vi "Reactor.vi"() -> ()   [LabVIEW 2017]
uses:
  <vilib>/Analysis/baseanly.llb/Mean (DBL).vi
  <vilib>/Utility/file.llb/Read Delimited Spreadsheet (DBL).vi
  <vilib>/Analysis/NI_AALBase.lvlib
panel:
  in  "CTAH Set Point":sgl format="%.1f"
  in  "Mode":string(combo)
  in  "Reset IHX Controller Mode":bool
  out "Server OK":bool
  out "System Time [s]":sgl
  out "Power Output":sgl(graph)
  out "Frequency [Hz]":sgl(slide) scale=0.0..60.0
  out "Frequency [Hz]":sgl(slide) scale=0.0..60.0
  out "Frequency [Hz]":sgl(knob) scale=0.0..45.0
  out "Power [W]":sgl(slide) caption="Power Output [W]" scale=0.0..10000.0
  in  "Desired Power [W]":dbl min=0.0 max=1000.0 step=1.0 format="%.1f"
  out "WT-10":sgl format="%.1f"
  out "BT-11":sgl format="%.1f"
  out "BT-12":sgl format="%.1f"
  out "WT-13":sgl format="%.1f"
  out "CX-10":dbl format="%.1f"
  out "CX-11":dbl format="%.1f"
  out "WT-20":sgl format="%.1f"
  out "BT-21":sgl format="%.1f"
  out "WT-22":sgl format="%.1f"
  out "BT-23":sgl format="%.1f"
  out "WT-24":sgl format="%.1f"
  out "BT-25":sgl format="%.1f"
  out "WT-26":sgl format="%.1f"
  out "BT-27":sgl format="%.1f"
  out "WT-28":sgl format="%.1f"
  out "BT-29":sgl format="%.1f"
  out "BT-30":sgl format="%.1f"
  out "WT-31":sgl format="%.1f"
  out "BT-32":sgl format="%.1f"
  out "WT-33":sgl format="%.1f"
  out "BT-34":sgl format="%.1f"
  out "WT-35":sgl format="%.1f"
  out "WT-40":sgl format="%.1f"
  out "BT-41":sgl format="%.1f"
  out "WT-42":sgl format="%.1f"
  out "BT-43":sgl format="%.1f"
  out "BT-60":sgl format="%.1f"
  out "WT-61":sgl format="%.1f"
  out "WT-62":sgl format="%.1f"
  out "BT-63":sgl format="%.1f"
  out "WT-64":sgl format="%.1f"
  out "BT-65":sgl format="%.1f"
  out "BT-66":sgl format="%.1f"
  out "WT-67":sgl format="%.1f"
  out "ST-10":sgl format="%.1f"
  out "ST-11":sgl format="%.1f"
  out "ST-12":sgl[](array[numeric]) format="%.1f"
  out "ST-13":sgl format="%.1f"
  out "ST-14":sgl[](array[numeric]) format="%.1f"
  out "AT-01":sgl format="%.1f"
  out "AT-02":sgl format="%.1f"
  in  "Power Output On":bool
  in  "ACTIVATE - CTAH":bool
  in  "ACTIVATE - TCHX":bool
  in  "TCHX Frequency [Hz]":sgl min=0 max=60 step=0.1 format="%.1f"
  in  "ACTIVATE - PUMP":bool
  in  "Pump Frequency [Hz]":sgl min=0 max=45 step=0.1 format="%.1f"
  out "DHX Primary Flow\n\n\nFM-20 [kg/s]":sgl format="%.3f"
  out "Bypass Flow\n\n\nFM-30 [kg/s]":sgl format="%.3f"
  out "Primary Flow\n\n\nFM-40 [kg/s]":sgl format="%.3f"
  out "DRACS Flow\n\n\nFM-60 [kg/s]":sgl format="%.3f"
  out "System Safe":bool
  in  "Exit Profile":bool
  in  "Select Operation Mode":T1(ring) caption="Select Operation Mode2"
  out "System Loop Time (ms)":u32
  in  "Load Power Profile":bool
  in  "Dyn. Power Profile File":path
  out "CTAH Temperatures":cluster{"CTAH Outlet":dbl, "CTAH Inlet":dbl}(graph)
  out "CTAH Outlet":dbl format="%0.2f"
  out "CTAH Inlet":dbl format="%0.2f"
  out "Core Temperatures":cluster{"Heater Inlet":dbl, "Heater Outlet":dbl}(graph)
  out "Heater Outlet":dbl format="%0.2f"
  out "Heater Inlet":dbl format="%0.2f"
  out "Profile Step":i32
  out "Power Input Signal [W]":dbl
  out "Output Current 2 [A]":dbl
  out "Output Voltage 2 [V]":dbl
  out "Output Current 1 [A]":dbl
  out "Output Voltage 1 [V]":dbl
  out "Loop Period [ms]":i64
  in  "Pump Operation Mode":i32(listbox)
  in  "TCHX Operation Mode":i32(listbox)
  in  "CTAH Operation Mode":i32(listbox)
  in  "Stop Reactor Interface":bool
  # "DRACS"
  # "PRIMARY"
  # "HOT DRACS"
  # "TCHX"
  # "HOT LEG"
  # "DHX TOP"
  # "N"
  # "COLD DRACS"
  # "DHX"
  # "E"
  # "S"
  # "W"
  # "BYPASS"
  # "N"
  # "CTAH"
  # "SE"
  # "SW"
  # "HEATER"
  # "DHX BOTTOM"
  # "COLD LEG"
  # "PUMP"
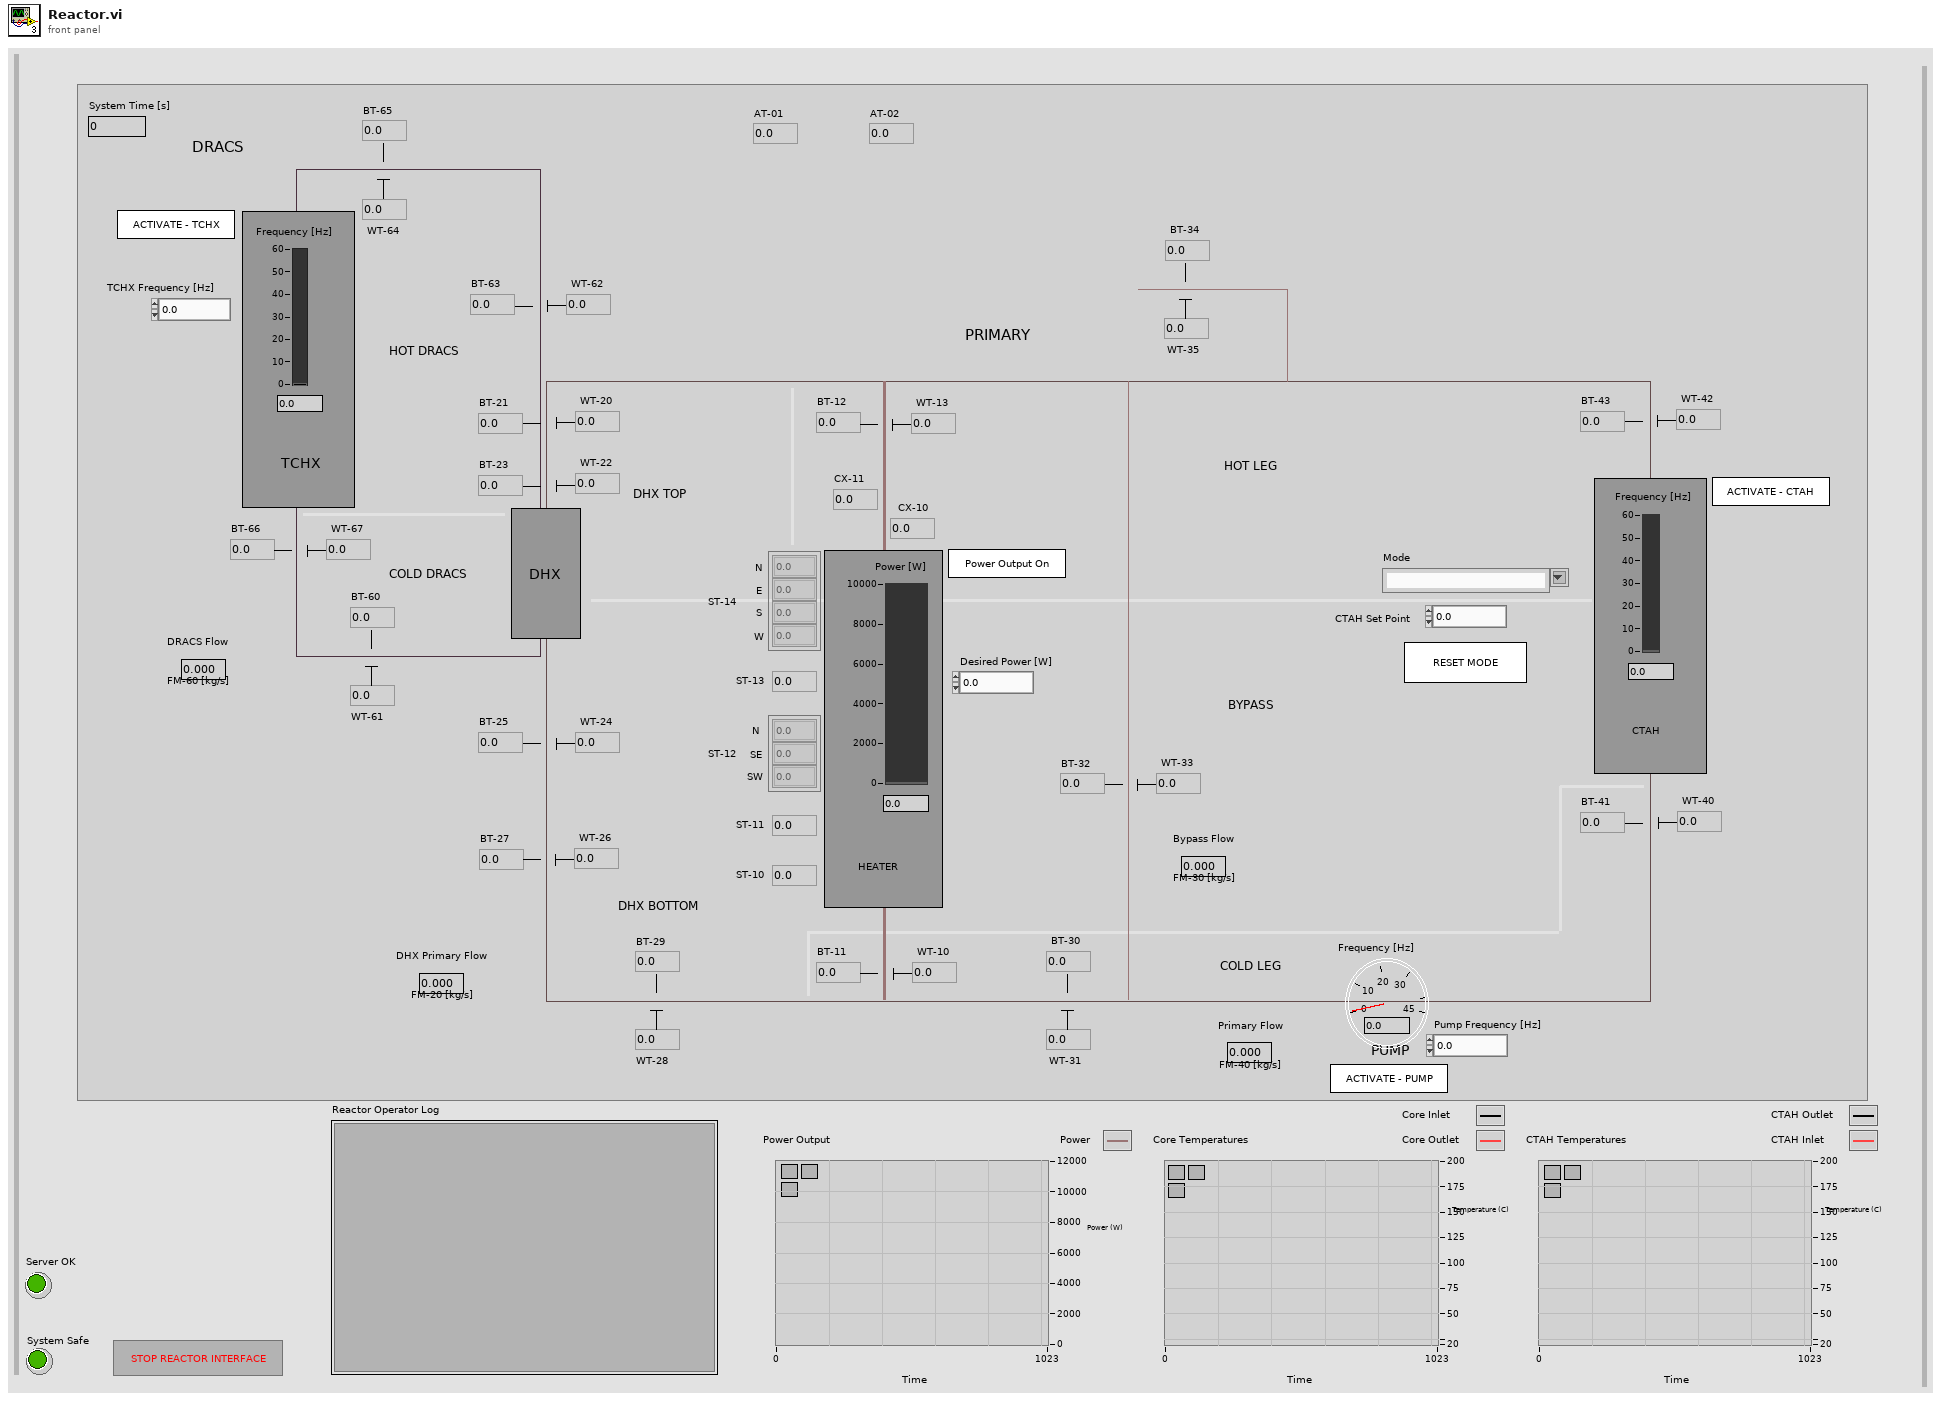
[diagram p1: front panel]
types:
  T1 = enum16{"Resistance Feedback", "Power Profile Input", "Resistance Feedback_Analog", "Power Profile Input_Analog", "Shutdown"}
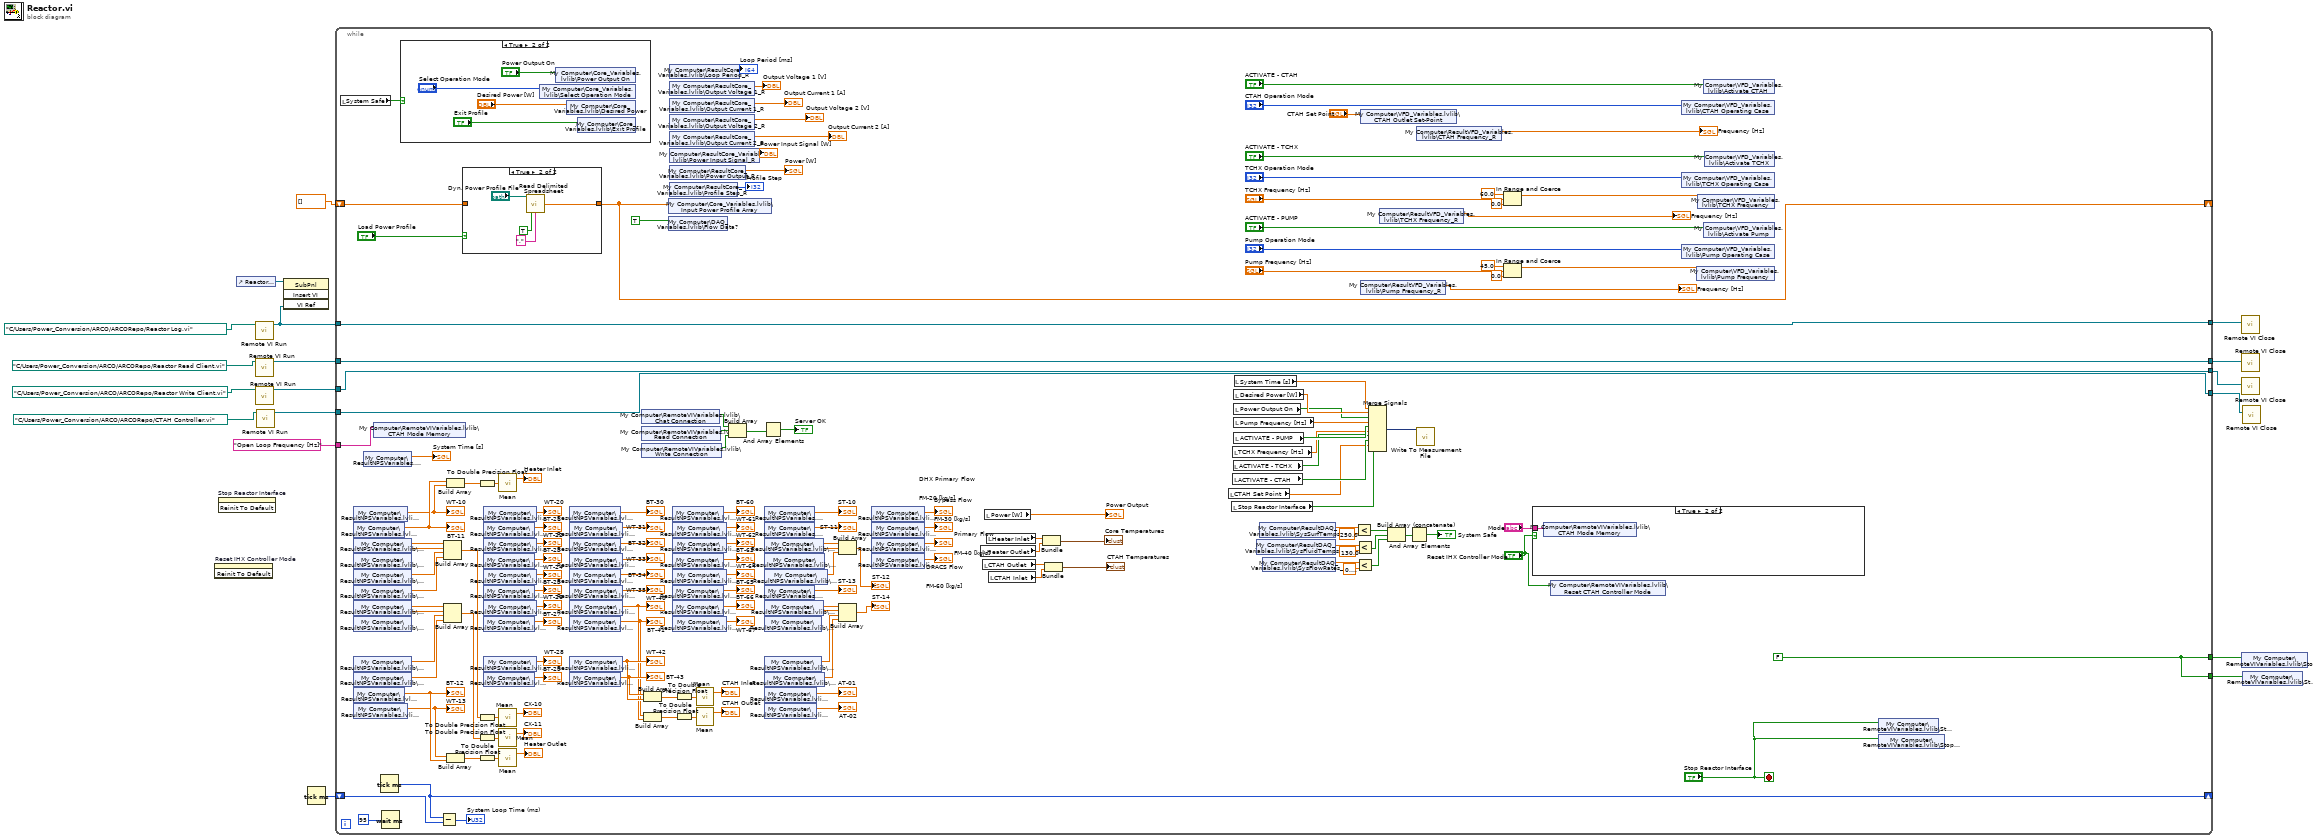
[diagram p0: block diagram]
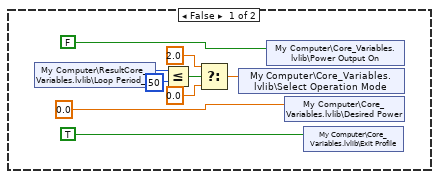
[diagram p3: hidden frame]
diagram:
  n1 = invoke on="Reset IHX Controller Mode" class="Bool" method="Reinit To Default"() -> ()  [unwired: 3 in, 3 out]
  n2 = invoke on="Stop Reactor Interface" class="Bool (strict)" method="Reinit To Default"() -> ()  [unwired: 3 in, 3 out]
  n3 = control-ref of="Reactor Operator Log"() -> (w12:refnum<vi>)
  n4 = call "Remote VI Run.vi"("VI Path"=path "C:/Users/Power_Conversion/ARCO/ARCORepo/Reactor Log.vi" ("vi path")) -> ("VI Reference"=w16:refnum<vi>)  [unwired: 10 in]
  n5 = call "Remote VI Run.vi"("VI Path"=path "C:/Users/Power_Conversion/ARCO/ARCORepo/Reactor Read Client.vi" ("vi path")) -> ("VI Reference"=w14:refnum<vi>)  [unwired: 10 in]
  n6 = call "Remote VI Run.vi"("VI Path"=path "C:/Users/Power_Conversion/ARCO/ARCORepo/Reactor Write Client.vi" ("vi path")) -> ("VI Reference"=w6:refnum<vi>)  [unwired: 10 in]
  n7 = call "Remote VI Run.vi"("VI Path"=path "C:/Users/Power_Conversion/ARCO/ARCORepo/CTAH Controller.vi" ("vi path")) -> ("VI Reference"=w3:refnum<vi>)  [unwired: 10 in]
  n8 = invoke on="Invoke Node" class="SubPnl" method="Insert VI"(reference=w12, "VI Ref"=w16) -> ()  [unwired: 2 in, 4 out]
  n9 = Tick Count (ms)() -> (millisecond timer value=w17:u32)
  n10 = while {
    shift-right: [w73] -> _
    shift-left: dbl[] [] ("Input Power Profile Array") -> [w74]
    shift-right: [w71] -> _
    shift-left: w17 -> [w72]
    tunnel: w16 -> [w53]
    tunnel: [w53] -> w15
    tunnel: w14 -> [w52]
    tunnel: [w52] -> w13
    tunnel: [w21] -> w11
    tunnel: "Open Loop Frequency [Hz]" -> [w20]
    tunnel: w6 -> [w26]
    tunnel: [w26] -> w5
    tunnel: w3 -> [w22]
    tunnel: [w22] -> w2
    tunnel: [w21] -> w1
    stop <- "Stop Reactor Interface" stop-if-true
    w21 = FALSE
    n11 = local read "System Safe"() -> (w57:bool)
    n12 = shared-variable "My Computer\\ResultNPSVariables.lvlib\\WT-10_R"() -> (w94:sgl)  [unwired: 1 in, 1 out]
    "WT-10" <- w94
    n13 = shared-variable "My Computer\\ResultNPSVariables.lvlib\\BT-11_R"() -> (w95:sgl)  [unwired: 1 in, 1 out]
    "BT-11" <- w95
    n14 = shared-variable "My Computer\\ResultNPSVariables.lvlib\\CX-10-1_R"() -> (w157:sgl)  [unwired: 1 in, 1 out]
    n15 = shared-variable "My Computer\\ResultNPSVariables.lvlib\\CX-10-2_R"() -> (w156:sgl)  [unwired: 1 in, 1 out]
    n16 = shared-variable "My Computer\\ResultNPSVariables.lvlib\\CX-10-3_R"() -> (w155:sgl)  [unwired: 1 in, 1 out]
    n17 = shared-variable "My Computer\\ResultNPSVariables.lvlib\\CX-10-4_R"() -> (w154:sgl)  [unwired: 1 in, 1 out]
    n18 = shared-variable "My Computer\\ResultNPSVariables.lvlib\\CX-11-1_R"() -> (w150:sgl)  [unwired: 1 in, 1 out]
    n19 = shared-variable "My Computer\\ResultNPSVariables.lvlib\\CX-11-2_R"() -> (w149:sgl)  [unwired: 1 in, 1 out]
    n20 = shared-variable "My Computer\\ResultNPSVariables.lvlib\\CX-11-3_R"() -> (w148:sgl)  [unwired: 1 in, 1 out]
    n21 = shared-variable "My Computer\\ResultNPSVariables.lvlib\\CX-11-4_R"() -> (w147:sgl)  [unwired: 1 in, 1 out]
    n22 = shared-variable "My Computer\\ResultNPSVariables.lvlib\\BT-12_R"() -> (w99:sgl)  [unwired: 1 in, 1 out]
    "BT-12" <- w99
    n23 = shared-variable "My Computer\\ResultNPSVariables.lvlib\\WT-13_R"() -> (w98:sgl)  [unwired: 1 in, 1 out]
    "WT-13" <- w98
    n24 = shared-variable "My Computer\\ResultNPSVariables.lvlib\\Time_R"() -> (→"System Time [s]":sgl)  [unwired: 1 in, 1 out]
    n25 = shared-variable "My Computer\\RemoteVIVariables.lvlib\\CTAH Mode Memory"(w20) -> ()  [unwired: 1 in, 1 out]
    n26 = Tick Count (ms)() -> (millisecond timer value=w71:u32)
    n27 = Wait (ms)(milliseconds to wait=u32 95) -> ()  [unwired: 1 out]
    n28 = case shown="True" w57 {
      frame False {
        n29 = shared-variable "My Computer\\ResultCore_Variables.lvlib\\Loop Period_R"() -> (w179:i64)  [unwired: 1 in, 1 out]
        n30 = Less Or Equal?(x=w179, y=i64 50) -> (x <= y?=w180:bool)
        n31 = Select(t=2.0, s=w180, f=0.0) -> (s? t:f=w175:dbl)
        n32 = shared-variable "My Computer\\Core_Variables.lvlib\\Select Operation Mode"(w175) -> ()  [unwired: 1 in, 1 out]
        n33 = shared-variable "My Computer\\Core_Variables.lvlib\\Power Output On"(FALSE ("Power Output On")) -> ()  [unwired: 1 in, 1 out]
        n34 = shared-variable "My Computer\\Core_Variables.lvlib\\Desired Power"(0.0 ("Desired Power")) -> ()  [unwired: 1 in, 1 out]
        n35 = shared-variable "My Computer\\Core_Variables.lvlib\\Exit Profile"(TRUE ("Exit Profile")) -> ()  [unwired: 1 in, 1 out]
      }
      frame True {
        n36 = shared-variable "My Computer\\Core_Variables.lvlib\\Select Operation Mode"("Select Operation Mode") -> ()  [unwired: 1 in, 1 out]
        n37 = shared-variable "My Computer\\Core_Variables.lvlib\\Power Output On"("Power Output On") -> ()  [unwired: 1 in, 1 out]
        n38 = shared-variable "My Computer\\Core_Variables.lvlib\\Desired Power"("Desired Power [W]") -> ()  [unwired: 1 in, 1 out]
        n39 = shared-variable "My Computer\\Core_Variables.lvlib\\Exit Profile"("Exit Profile") -> ()  [unwired: 1 in, 1 out]
      }
    }
    n40 = Subtract(x=w71, y=w72) -> (x-y=→"System Loop Time (ms)":u32)
    n41 = Build Array(w157, w156, w155, w154) -> (w153:sgl[])
    n42 = Build Array(w150, w149, w148, w147) -> (w146:sgl[])
    n43 = Build Array(w95, w94) -> (w96:sgl[])
    n44 = Build Array(w98, w99) -> (w100:sgl[])
    n45 = case shown="True" "Load Power Profile" {
      tunnel: [w188 w189] -> w73
      tunnel: w74 -> [w188 _]
      frame False {
      }
      frame True {
        n46 = call-poly <vilib>:"Read Delimited Spreadsheet.vi"("file path (dialog if empty)"="Dyn. Power Profile File", "transpose? (F)"=TRUE, "delimiter (\\t)"="," ("delimiter (\\t)")) -> ("first row"=w189:dbl[])  [unwired: 7 in, 5 out]
      }
    }
    n47 = To Double Precision Float(number=w96) -> (double precision float=w97:dbl[])
    n48 = To Double Precision Float(number=w153) -> (double precision float=w152:dbl[])
    n49 = To Double Precision Float(number=w146) -> (double precision float=w151:dbl[])
    n50 = To Double Precision Float(number=w100) -> (double precision float=w101:dbl[])
    n51 = shared-variable "My Computer\\ResultNPSVariables.lvlib\\WT-20_R"() -> (→"WT-20":sgl)  [unwired: 1 in, 1 out]
    n52 = shared-variable "My Computer\\ResultNPSVariables.lvlib\\BT-21_R"() -> (→"BT-21":sgl)  [unwired: 1 in, 1 out]
    n53 = shared-variable "My Computer\\ResultNPSVariables.lvlib\\WT-22_R"() -> (→"WT-22":sgl)  [unwired: 1 in, 1 out]
    n54 = shared-variable "My Computer\\ResultNPSVariables.lvlib\\BT-23_R"() -> (→"BT-23":sgl)  [unwired: 1 in, 1 out]
    n55 = shared-variable "My Computer\\ResultNPSVariables.lvlib\\WT-24_R"() -> (→"WT-24":sgl)  [unwired: 1 in, 1 out]
    n56 = shared-variable "My Computer\\ResultNPSVariables.lvlib\\BT-25_R"() -> (→"BT-25":sgl)  [unwired: 1 in, 1 out]
    n57 = shared-variable "My Computer\\ResultNPSVariables.lvlib\\WT-26_R"() -> (→"WT-26":sgl)  [unwired: 1 in, 1 out]
    n58 = shared-variable "My Computer\\ResultNPSVariables.lvlib\\BT-27_R"() -> (→"BT-27":sgl)  [unwired: 1 in, 1 out]
    n59 = shared-variable "My Computer\\ResultNPSVariables.lvlib\\WT-28_R"() -> (→"WT-28":sgl)  [unwired: 1 in, 1 out]
    n60 = shared-variable "My Computer\\ResultNPSVariables.lvlib\\BT-29_R"() -> (→"BT-29":sgl)  [unwired: 1 in, 1 out]
    n61 = call-poly <vilib>:"Mean.vi"("X"=w97) -> ("mean"=→"Heater Inlet":dbl)  [unwired: 1 out]
    n62 = call-poly <vilib>:"Mean.vi"("X"=w152) -> ("mean"=→"CX-10":dbl)  [unwired: 1 out]
    n63 = call-poly <vilib>:"Mean.vi"("X"=w151) -> ("mean"=→"CX-11":dbl)  [unwired: 1 out]
    n64 = call-poly <vilib>:"Mean.vi"("X"=w101) -> ("mean"=→"Heater Outlet":dbl)  [unwired: 1 out]
    n65 = shared-variable "My Computer\\ResultNPSVariables.lvlib\\BT-30_R"() -> (→"BT-30":sgl)  [unwired: 1 in, 1 out]
    n66 = shared-variable "My Computer\\ResultNPSVariables.lvlib\\WT-31_R"() -> (→"WT-31":sgl)  [unwired: 1 in, 1 out]
    n67 = shared-variable "My Computer\\ResultNPSVariables.lvlib\\BT-32_R"() -> (→"BT-32":sgl)  [unwired: 1 in, 1 out]
    n68 = shared-variable "My Computer\\ResultNPSVariables.lvlib\\WT-33_R"() -> (→"WT-33":sgl)  [unwired: 1 in, 1 out]
    n69 = shared-variable "My Computer\\ResultNPSVariables.lvlib\\BT-34_R"() -> (→"BT-34":sgl)  [unwired: 1 in, 1 out]
    n70 = shared-variable "My Computer\\ResultNPSVariables.lvlib\\WT-35_R"() -> (→"WT-35":sgl)  [unwired: 1 in, 1 out]
    n71 = shared-variable "My Computer\\ResultNPSVariables.lvlib\\WT-40_R"() -> (w80:sgl)  [unwired: 1 in, 1 out]
    "WT-40" <- w80
    n72 = shared-variable "My Computer\\ResultNPSVariables.lvlib\\BT-41_R"() -> (w79:sgl)  [unwired: 1 in, 1 out]
    "BT-41" <- w79
    n73 = shared-variable "My Computer\\ResultNPSVariables.lvlib\\WT-42_R"() -> (w82:sgl)  [unwired: 1 in, 1 out]
    "WT-42" <- w82
    n74 = shared-variable "My Computer\\ResultNPSVariables.lvlib\\BT-43_R"() -> (w81:sgl)  [unwired: 1 in, 1 out]
    "BT-43" <- w81
    n75 = shared-variable "My Computer\\RemoteVIVariables.lvlib\\Chat Connection"() -> (w51:bool)  [unwired: 1 in, 1 out]
    n76 = shared-variable "My Computer\\RemoteVIVariables.lvlib\\Read Connection"() -> (w50:bool)  [unwired: 1 in, 1 out]
    n77 = shared-variable "My Computer\\RemoteVIVariables.lvlib\\Write Connection"() -> (w25:bool)  [unwired: 1 in, 1 out]
    n78 = Build Array(w81, w82) -> (w87:sgl[])
    n79 = Build Array(w79, w80) -> (w84:sgl[])
    n80 = shared-variable "My Computer\\Core_Variables.lvlib\\Input Power Profile Array"(w73) -> ()  [unwired: 1 in, 1 out]
    n81 = shared-variable "My Computer\\DAQ_Variables.lvlib\\Flow Data?"(TRUE ("Flow Data?")) -> ()  [unwired: 1 in, 1 out]
    n82 = shared-variable "My Computer\\ResultCore_Variables.lvlib\\Loop Period_R"() -> (→"Loop Period [ms]":i64)  [unwired: 1 in, 1 out]
    n83 = shared-variable "My Computer\\ResultCore_Variables.lvlib\\Output Voltage 1_R"() -> (→"Output Voltage 1 [V]":dbl)  [unwired: 1 in, 1 out]
    n84 = shared-variable "My Computer\\ResultCore_Variables.lvlib\\Output Current 1_R"() -> (→"Output Current 1 [A]":dbl)  [unwired: 1 in, 1 out]
    n85 = shared-variable "My Computer\\ResultCore_Variables.lvlib\\Output Voltage 2_R"() -> (→"Output Voltage 2 [V]":dbl)  [unwired: 1 in, 1 out]
    n86 = shared-variable "My Computer\\ResultCore_Variables.lvlib\\Output Current 2_R"() -> (→"Output Current 2 [A]":dbl)  [unwired: 1 in, 1 out]
    n87 = shared-variable "My Computer\\ResultCore_Variables.lvlib\\Power Input Signal_R"() -> (→"Power Input Signal [W]":sgl)  [unwired: 1 in, 1 out]
    n88 = shared-variable "My Computer\\ResultCore_Variables.lvlib\\Power Output_R"() -> (→"Power [W]":sgl)  [unwired: 1 in, 1 out]
    n89 = shared-variable "My Computer\\ResultCore_Variables.lvlib\\Profile Step_R"() -> (→"Profile Step":i32)  [unwired: 1 in, 1 out]
    n90 = shared-variable "My Computer\\ResultNPSVariables.lvlib\\BT-60_R"() -> (→"BT-60":sgl)  [unwired: 1 in, 1 out]
    n91 = shared-variable "My Computer\\ResultNPSVariables.lvlib\\WT-61_R"() -> (→"WT-61":sgl)  [unwired: 1 in, 1 out]
    n92 = shared-variable "My Computer\\ResultNPSVariables.lvlib\\WT-62_R"() -> (→"WT-62":sgl)  [unwired: 1 in, 1 out]
    n93 = shared-variable "My Computer\\ResultNPSVariables.lvlib\\BT-63_R"() -> (→"BT-63":sgl)  [unwired: 1 in, 1 out]
    n94 = shared-variable "My Computer\\ResultNPSVariables.lvlib\\WT-64_R"() -> (→"WT-64":sgl)  [unwired: 1 in, 1 out]
    n95 = shared-variable "My Computer\\ResultNPSVariables.lvlib\\BT-65_R"() -> (→"BT-65":sgl)  [unwired: 1 in, 1 out]
    n96 = shared-variable "My Computer\\ResultNPSVariables.lvlib\\BT-66_R"() -> (→"BT-66":sgl)  [unwired: 1 in, 1 out]
    n97 = shared-variable "My Computer\\ResultNPSVariables.lvlib\\WT-67_R"() -> (→"WT-67":sgl)  [unwired: 1 in, 1 out]
    n98 = To Double Precision Float(number=w87) -> (double precision float=w88:dbl[])
    n99 = To Double Precision Float(number=w84) -> (double precision float=w85:dbl[])
    n100 = call-poly <vilib>:"Mean.vi"("X"=w88) -> ("mean"=→"CTAH Inlet":dbl)  [unwired: 1 out]
    n101 = call-poly <vilib>:"Mean.vi"("X"=w85) -> ("mean"=→"CTAH Outlet":dbl)  [unwired: 1 out]
    n102 = Build Array(w51, w50, w25) -> (w49:bool[])
    n103 = And Array Elements(Boolean array=w49) -> (logical AND=→"Server OK":bool)
    n104 = shared-variable "My Computer\\ResultNPSVariables.lvlib\\ST-10_R"() -> (→"ST-10":sgl)  [unwired: 1 in, 1 out]
    n105 = shared-variable "My Computer\\ResultNPSVariables.lvlib\\ST-11_R"() -> (→"ST-11":sgl)  [unwired: 1 in, 1 out]
    n106 = shared-variable "My Computer\\ResultNPSVariables.lvlib\\ST-12-N_R"() -> (w117:sgl)  [unwired: 1 in, 1 out]
    n107 = shared-variable "My Computer\\ResultNPSVariables.lvlib\\ST-12-SE_R"() -> (w116:sgl)  [unwired: 1 in, 1 out]
    n108 = shared-variable "My Computer\\ResultNPSVariables.lvlib\\ST-12-SW_R"() -> (w115:sgl)  [unwired: 1 in, 1 out]
    n109 = shared-variable "My Computer\\ResultNPSVariables.lvlib\\ST-13_R"() -> (→"ST-13":sgl)  [unwired: 1 in, 1 out]
    n110 = shared-variable "My Computer\\ResultNPSVariables.lvlib\\ST-14-N_R"() -> (w112:sgl)  [unwired: 1 in, 1 out]
    n111 = shared-variable "My Computer\\ResultNPSVariables.lvlib\\ST-14-E_R"() -> (w111:sgl)  [unwired: 1 in, 1 out]
    n112 = shared-variable "My Computer\\ResultNPSVariables.lvlib\\ST-14-S_R"() -> (w110:sgl)  [unwired: 1 in, 1 out]
    n113 = shared-variable "My Computer\\ResultNPSVariables.lvlib\\ST-14-W_R"() -> (w109:sgl)  [unwired: 1 in, 1 out]
    n114 = shared-variable "My Computer\\ResultNPSVariables.lvlib\\AT-01_R"() -> (→"AT-01":sgl)  [unwired: 1 in, 1 out]
    n115 = shared-variable "My Computer\\ResultNPSVariables.lvlib\\AT-02_R"() -> (→"AT-02":sgl)  [unwired: 1 in, 1 out]
    n116 = Build Array(w117, w116, w115) -> (→"ST-12":sgl[])
    n117 = Build Array(w112, w111, w110, w109) -> (→"ST-14":sgl[])
    n118 = shared-variable "My Computer\\ResultNPSVariables.lvlib\\FM-20_R"() -> (→"DHX Primary Flow\n\n\nFM-20 [kg/s]":sgl)  [unwired: 1 in, 1 out]
    n119 = shared-variable "My Computer\\ResultNPSVariables.lvlib\\FM-30_R"() -> (→"Bypass Flow\n\n\nFM-30 [kg/s]":sgl)  [unwired: 1 in, 1 out]
    n120 = shared-variable "My Computer\\ResultNPSVariables.lvlib\\FM-40_R"() -> (→"Primary Flow\n\n\nFM-40 [kg/s]":sgl)  [unwired: 1 in, 1 out]
    n121 = shared-variable "My Computer\\ResultNPSVariables.lvlib\\FM-60_R"() -> (→"DRACS Flow\n\n\nFM-60 [kg/s]":sgl)  [unwired: 1 in, 1 out]
    n122 = local read "Heater Outlet"() -> (w89:dbl)
    n123 = local read "CTAH Outlet"() -> (w77:dbl)
    n124 = local read "Power [W]"() -> (→"Power Output":sgl)
    n125 = local read "Heater Inlet"() -> (w90:dbl)
    n126 = local read "CTAH Inlet"() -> (w76:dbl)
    n127 = Bundle("Heater Inlet"=w90, "Heater Outlet"=w89) -> (→"Core Temperatures":cluster{"Heater Inlet":dbl, "Heater Outlet":dbl})  [unwired: 1 in]
    n128 = Bundle("CTAH Outlet"=w77, "CTAH Inlet"=w76) -> (→"CTAH Temperatures":cluster{"CTAH Outlet":dbl, "CTAH Inlet":dbl})  [unwired: 1 in]
    n129 = local read "CTAH Set Point"() -> (w29:sgl)
    n130 = local read "Stop Reactor Interface"() -> (w28:bool)
    n131 = local read "TCHX Frequency [Hz]"() -> (w32:sgl)
    n132 = local read "ACTIVATE - CTAH"() -> (w30:bool)
    n133 = local read "ACTIVATE - TCHX"() -> (w31:bool)
    n134 = local read "Desired Power [W]"() -> (w36:dbl)
    n135 = local read "Power Output On"() -> (w35:bool)
    n136 = local read "Pump Frequency [Hz]"() -> (w34:sgl)
    n137 = local read "ACTIVATE - PUMP"() -> (w33:bool)
    n138 = local read "System Time [s]"() -> (w37:sgl)
    n139 = shared-variable "My Computer\\ResultDAQ_Variables.lvlib\\SysFluidTemps_R"() -> (w63:sgl[])  [unwired: 1 in, 1 out]
    n140 = shared-variable "My Computer\\ResultDAQ_Variables.lvlib\\SysSurfTemps_R"() -> (w65:sgl[])  [unwired: 1 in, 1 out]
    n141 = shared-variable "My Computer\\ResultDAQ_Variables.lvlib\\SysFlowRates_R"() -> (w61:sgl[])  [unwired: 1 in, 1 out]
    n142 = Less?(x=w65, y=sgl 250.0) -> (x < y?=w67:bool[])
    n143 = Less?(x=w63, y=sgl 130.0) -> (x < y?=w60:bool[])
    n144 = Less?(x=w61, y=sgl 0.2) -> (x < y?=w59:bool[])
    n145 = shared-variable "My Computer\\VFD_Variables.lvlib\\CTAH Outlet Set-Point"("CTAH Set Point") -> ()  [unwired: 1 in, 1 out]
    n146 = shared-variable "My Computer\\ResultVFD_Variables.lvlib\\Pump Frequency_R"() -> (→"Frequency [Hz]":sgl)  [unwired: 1 in, 1 out]
    n147 = Merge Signals(w37, w36, w35, w34, w33, w32, w31, w30, w29, w28) -> (w38:dynamicdata)
    n148 = shared-variable "My Computer\\ResultVFD_Variables.lvlib\\TCHX Frequency_R"() -> (→"Frequency [Hz]":sgl)  [unwired: 1 in, 1 out]
    n149 = Build Array (concatenate)(w67, w60, w59) -> (w68:bool[])
    n150 = And Array Elements(Boolean array=w68) -> (logical AND=→"System Safe":bool)
    n151 = shared-variable "My Computer\\ResultVFD_Variables.lvlib\\CTAH Frequency_R"() -> (→"Frequency [Hz]":sgl)  [unwired: 1 in, 1 out]
    n152 = call "Write To Measurement File"("Signals"=w38) -> ()  [unwired: 16 in, 3 out]
    n153 = In Range and Coerce(upper limit=sgl 60.0, x="TCHX Frequency [Hz]", lower limit=sgl 0.0) -> (coerced(x)=w43:sgl)  [unwired: 1 out]
    n154 = In Range and Coerce(upper limit=sgl 45.0, x="Pump Frequency [Hz]", lower limit=sgl 0.0) -> (coerced(x)=w42:sgl)  [unwired: 1 out]
    n155 = case shown="True" "Reset IHX Controller Mode" {
      tunnel: "Mode" -> [_ w174]
      frame False {
      }
      frame True {
        n156 = shared-variable "My Computer\\RemoteVIVariables.lvlib\\CTAH Mode Memory"(w174) -> ()  [unwired: 1 in, 1 out]
      }
    }
    n157 = shared-variable "My Computer\\RemoteVIVariables.lvlib\\Reset CTAH Controller Mode"("Reset IHX Controller Mode") -> ()  [unwired: 1 in, 1 out]
    n158 = shared-variable "My Computer\\VFD_Variables.lvlib\\CTAH Operating Case"("CTAH Operation Mode") -> ()  [unwired: 1 in, 1 out]
    n159 = shared-variable "My Computer\\VFD_Variables.lvlib\\Pump Operating Case"("Pump Operation Mode") -> ()  [unwired: 1 in, 1 out]
    n160 = shared-variable "My Computer\\VFD_Variables.lvlib\\TCHX Operating Case"("TCHX Operation Mode") -> ()  [unwired: 1 in, 1 out]
    n161 = shared-variable "My Computer\\VFD_Variables.lvlib\\Pump Frequency"(w42) -> ()  [unwired: 1 in, 1 out]
    n162 = shared-variable "My Computer\\VFD_Variables.lvlib\\TCHX Frequency"(w43) -> ()  [unwired: 1 in, 1 out]
    n163 = shared-variable "My Computer\\VFD_Variables.lvlib\\Activate CTAH"("ACTIVATE - CTAH") -> ()  [unwired: 1 in, 1 out]
    n164 = shared-variable "My Computer\\VFD_Variables.lvlib\\Activate Pump"("ACTIVATE - PUMP") -> ()  [unwired: 1 in, 1 out]
    n165 = shared-variable "My Computer\\VFD_Variables.lvlib\\Activate TCHX"("ACTIVATE - TCHX") -> ()  [unwired: 1 in, 1 out]
    n166 = shared-variable "My Computer\\RemoteVIVariables.lvlib\\Stop CTAH"("Stop Reactor Interface") -> ()  [unwired: 1 in, 1 out]
    n167 = shared-variable "My Computer\\RemoteVIVariables.lvlib\\Stop Reading"("Stop Reactor Interface") -> ()  [unwired: 1 in, 1 out]
  }
  n168 = call "Remote VI Close.vi"("reference"=w15) -> ()  [unwired: 10 in, 1 out]
  n169 = call "Remote VI Close.vi"("reference"=w13) -> ()  [unwired: 10 in, 1 out]
  n170 = shared-variable "My Computer\\RemoteVIVariables.lvlib\\Stop Reading"(w11) -> ()  [unwired: 1 in, 1 out]
  n171 = call "Remote VI Close.vi"("reference"=w5) -> ()  [unwired: 10 in, 1 out]
  n172 = call "Remote VI Close.vi"("reference"=w2) -> ()  [unwired: 10 in, 1 out]
  n173 = shared-variable "My Computer\\RemoteVIVariables.lvlib\\Stop CTAH"(w1) -> ()  [unwired: 1 in, 1 out]
